vi "VNA_Close.vi"(7 "HAPS_MCU_CMD":enum16{"Keysight", "R&S"}(ring), 8 "error in":errorcluster) -> (0 "error out":errorcluster)   [LabVIEW 2023, in "HAPS.lvlib"]
uses:
  HAPS.lvlib
  CTL/Keysight_VNA.ctl
  CTL/RS_ZNA.ctl
  Keysight/Keysight.lvlib
  R_S/R_S.lvlib
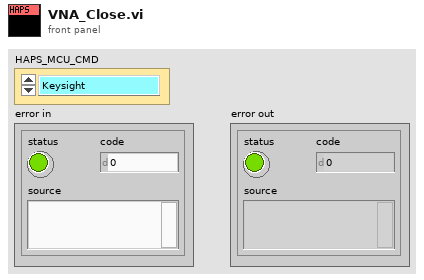
[diagram p1: front panel]
types:
  T1 = typedef "Keysight_VNA.ctl" = enum16{"Init", "queryMarker", "setSweepPoint", "setMarkerFreq", "setMeasureFormat", "setFreqStartStop", "setMarkerOnOFF", "setMarkerFormat_LOGP", "setMeasPAR_S", "setTriggerSingle", "Trigger_Save_SnP", "Trigger_Single", "Close"}
  T2 = typedef "RS_ZNA.ctl" = enum16{"Init", "Close", "set_SweepPoint", "set_MeasFormat", "set_FreqStartStop", "set_MeasPAR_S", "set_MarkerON", "set_MarkerOFF", "set_MarkerFreq", "set_MarkerFormat", "set_TriggerSingle", "query_GainPhase"}
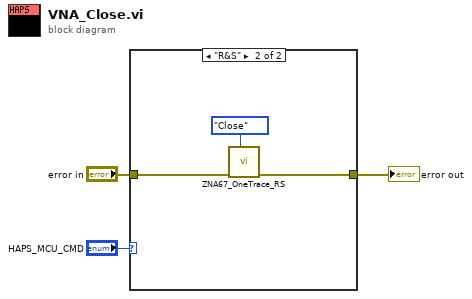
[diagram p0: block diagram]
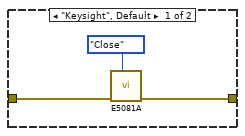
[diagram p2: hidden frame]
diagram:
  n1 = case shown="\"R&S\"" "HAPS_MCU_CMD" {
    tunnel: "error in" -> [w6 w8]
    tunnel: [w5 w9] -> w1
    frame "Keysight", Default {
      n2 = call "E5081A.vi"("Function_VNA"=Keysight_VNA."Close", "error in"=w6) -> ("error out"=w5:errorcluster)  [unwired: 8 in, 1 out]
    }
    frame "R&S" {
      n3 = call "ZNA67_OneTrace_RS.vi"("ZNA_Func."=RS_ZNA."Close", "error in"=w8) -> ("error out"=w9:errorcluster)  [unwired: 6 in, 3 out]
    }
  }
  "error out" <- w1
